vi "test_UDP_Open connection using Initialize node.vi"(8 "error in (no error)":errorcluster, 11 "TestCase in":refnum<class "Ethernet Protocol Tests.lvclass">) -> (0 "error out":errorcluster, 3 "TestCase out":refnum<class "Ethernet Protocol Tests.lvclass">)   [LabVIEW 2019, in "Ethernet Protocol Tests.lvclass"]
uses:
  Ethernet Protocol Tests.lvclass
  UDP/UDP.lvclass
  UDP/UDP.lvclass/UDP.ctl
  UDP/Data Access/Write Local IP Address.vi
  UDP/Data Access/Write Target IP Address.vi
  UDP/Data Access/Write Local Port.vi
  UDP/Data Access/Write Target Port.vi
  <vilib>/addons/_JKI Toolkits/VI Tester/TestCase.llb/TestCase.lvclass
  C:/Program Files (x86)/National Instruments/LabVIEW 2019/vi.lib/addons/_JKI Toolkits/VI Tester/TestCase.llb/TestCase.lvclass
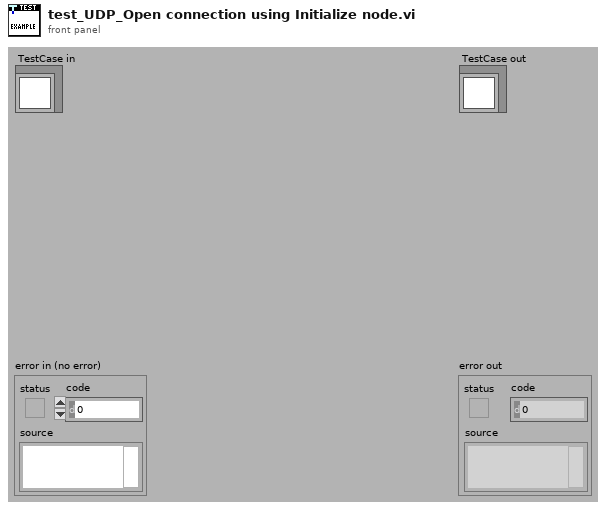
[diagram p1: front panel]
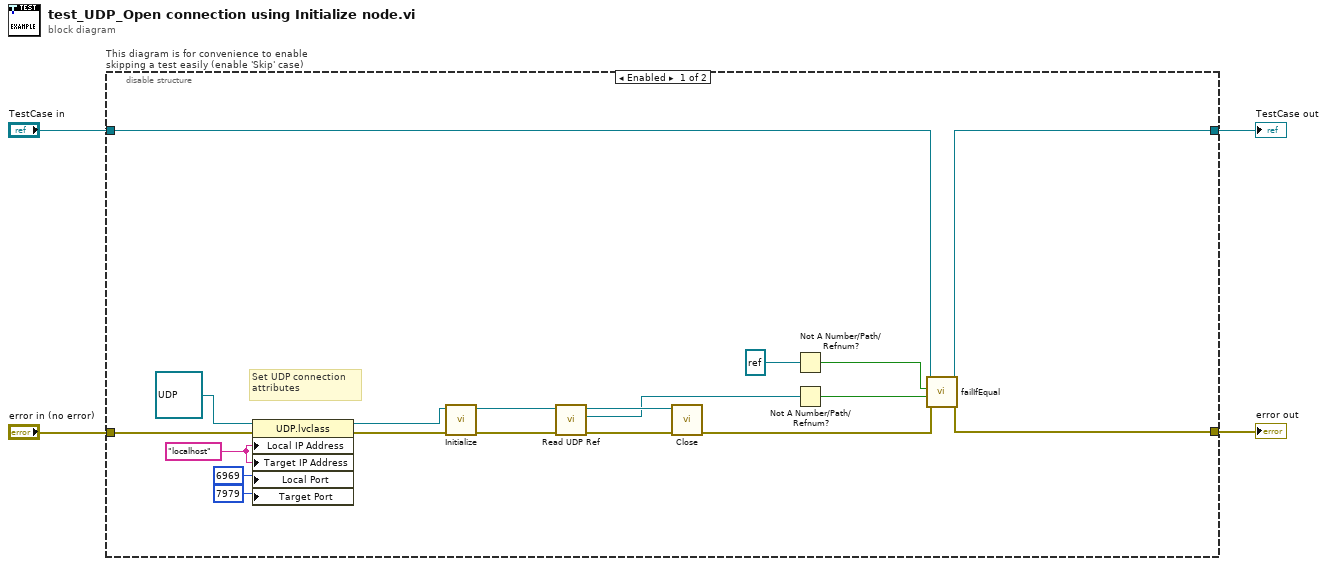
[diagram p0: block diagram]
diagram:
  n1 = disable-structure "This diagram is for convenience to enable skipping a test easily (enable 'Skip' case)" shown="Enabled" {
    disable-tunnel: "TestCase in" -> [w23 w27]
    disable-tunnel: [w22 w25] -> w1
    disable-tunnel: [w21 w26] -> w3
    disable-tunnel: "error in (no error)" -> [w19 w24]
    frame Enabled {
      w18 = "localhost" ("Local IP Address")
      # "Set UDP connection \nattributes"
      n2 = property class="UDP.lvclass"(reference=refnum<class "UDP.lvclass"> refnum ("Protocols.lvlib:UDP.lvclass"), error in=w19, "Local IP Address"=w18, "Target IP Address"=w18, "Local Port"=u16 6969, "Target Port"=u16 7979) -> (reference out=w7:refnum<class "UDP.lvclass">, error out=w8:errorcluster)
      n3 = call-dynamic "Initialize.vi"("error in (no error)"=w8, "UDP in"=w7) -> ("error out"=w6:errorcluster, "UDP out"=w5:refnum<class "UDP.lvclass">)  [unwired: 8 in]
      n4 = call "Read UDP Ref.vi"("error in (no error)"=w6, "UDP in"=w5) -> ("error out"=w14:errorcluster, "UDP Ref"=w12:refnum<k16>, "UDP out"=w13:refnum<class "UDP.lvclass">)  [unwired: 7 in]
      n5 = call-dynamic "Close.vi"("error in (no error)"=w14, "UDP in"=w13) -> ("error out"=w15:errorcluster)  [unwired: 8 in, 1 out]
      n6 = Not A Number/Path/Refnum?(number/path/refnum=refnum<k16> refnum ("UDP Ref")) -> (NaN/Path/Refnum?=w9:bool)
      n7 = Not A Number/Path/Refnum?(number/path/refnum=w12) -> (NaN/Path/Refnum?=w11:bool)
      n8 = call-dynamic "failIfEqual.vi"("error in (no error)"=w15, "y"=w11, "x"=w9, "TestCase in"=w23) -> ("error out"=w21:errorcluster, "TestCase out"=w22:refnum<class "Ethernet Protocol Tests.lvclass">)  [unwired: 6 in]
    }
    frame Disabled {
      # "skip test result while test is under development"
      n9 = call <vilib>:"skip.vi"("error in (no error)"=w24, "TestCase in"=w27) -> ("error out"=w26:errorcluster, "TestCase out"=w25:refnum<class "Ethernet Protocol Tests.lvclass">)  [unwired: 8 in]
    }
  }
  "error out" <- w3
  "TestCase out" <- w1
